vi "PulseGeneratorSetup.vi"(4 "Pulse duration (s)\nif more than one pulse":dbl, 5 "Channel":enum16{"1", "2", "3", "4", "5", "6", "7", "8"}(ring), 6 "Pulses per\nstimulus":u16, 7 "stimulus specifier":T3, 8 "Stimulus\nduration (s)":dbl, 9 "Time between stimuli,\nstart-to-start (s)":dbl, 10 "Number\nof stimuli":u16, 11 "Initial delay (s)":dbl) -> (0 "error IO":errorcluster, 1 "stimulus parameters":T1, 2 "stimulus information":T2, 3 "stimulus specifier":T3)   [LabVIEW 2014]
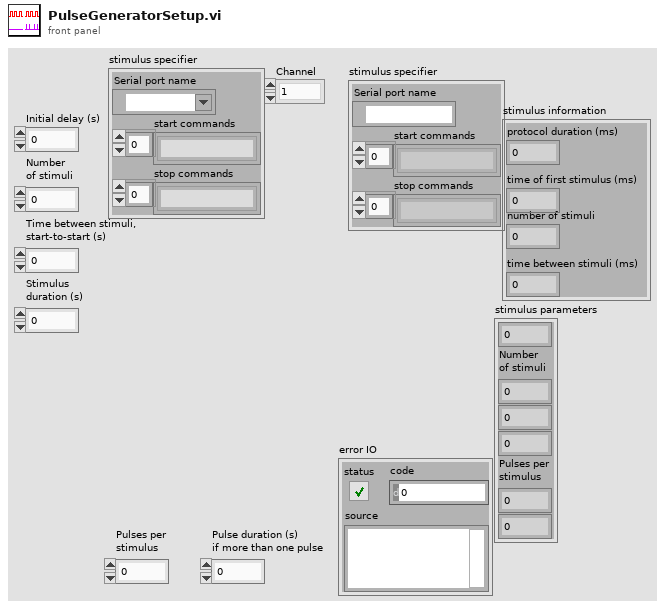
[diagram p1: front panel]
types:
  T1 = cluster{dbl, "Number\nof stimuli":u16, dbl, dbl, "Pulses per\nstimulus":u16, dbl}
  T2 = cluster{"protocol duration (ms)":i64, "time of first stimulus (ms)":i64, "number of stimuli":u16, "time between stimuli (ms)":i64}
  T3 = cluster{"Serial port name":refnum<visa-resource-name>, "start commands":string[], "stop commands":string[]}
  T4 = cluster{i64, "result (ms)":i64, "Number\nof stimuli":u16, i64}
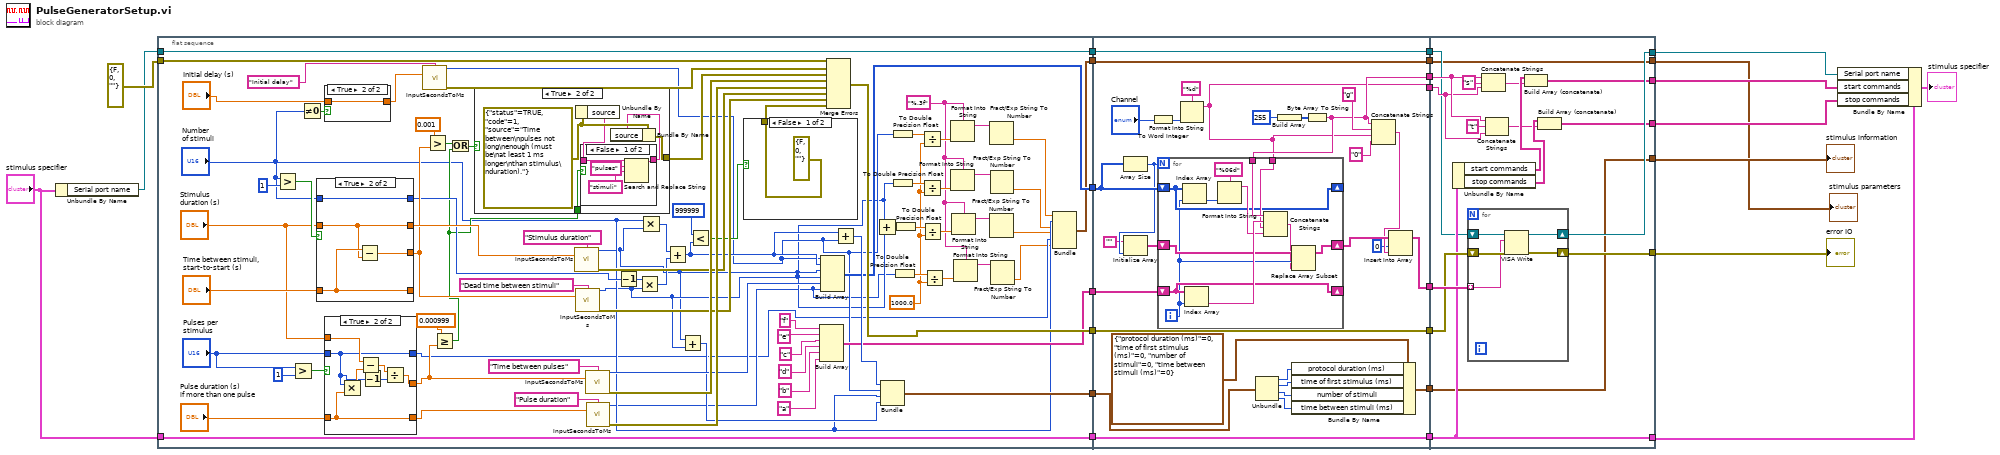
[diagram p0: block diagram]
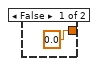
[diagram p2: hidden frame]
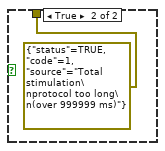
[diagram p3: hidden frame]
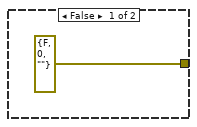
[diagram p4: hidden frame]
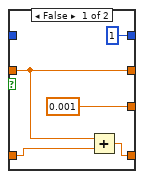
[diagram p6: hidden frame]
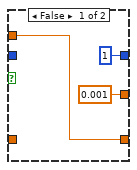
[diagram p7: hidden frame]
diagram:
  n1 = Unbundle By Name("stimulus specifier") -> ("Serial port name"=w11:refnum<visa-resource-name>)
  n2 = flat-sequence {
    tunnel: [w53] -> w9
    tunnel: [w54] -> w8
    tunnel: [w71] -> w7
    tunnel: [w69] -> w6
    tunnel: [w66] -> w5
    tunnel: "stimulus specifier" -> [w69]
    tunnel: errorcluster {"status"=FALSE, "code"=0, "source"=""} ("error constant") -> [w56]
    tunnel: w11 -> [w55]
    tunnel: [w55] -> w4
    tunnel: [w27] -> w3
    tunnel: w9 -> [w169]
    tunnel: w8 -> [w168]
    tunnel: w7 -> [w154]
    tunnel: [w155] -> w26
    tunnel: [w154] -> w25
    tunnel: [w153] -> w24
    tunnel: [w152] -> w23
    tunnel: w6 -> [w151]
    tunnel: [w151] -> w21
    tunnel: w5 -> [w149]
    tunnel: [w144] -> w15
    tunnel: w4 -> [w143]
    tunnel: [w143] -> w10
    tunnel: w3 -> [w142]
    tunnel: [w142] -> w2
    tunnel: w26 -> [w200]
    tunnel: w25 -> [w199]
    tunnel: w24 -> [w196]
    tunnel: w23 -> [w195]
    tunnel: [w194] -> w22
    tunnel: w21 -> [w186]
    tunnel: [w193] -> w19
    tunnel: [w188] -> w18
    tunnel: [w187] -> w17
    tunnel: [w186] -> w20
    tunnel: w15 -> [w185]
    tunnel: [w185] -> w14
    tunnel: w10 -> [w184]
    tunnel: w2 -> [w183]
    tunnel: [w183] -> w1
    frame #0 {
      w40 = 1000.0 ("default (0 I32)")
      w39 = "%.3f"
      n3 = Greater?(x="Number\nof stimuli", y=u16 1) -> (0:w102:bool)
      n4 = Greater?(x="Pulses per\nstimulus", y=u16 1) -> (0:w107:bool)
      n5 = Not Equal To 0?(x="Number\nof stimuli") -> (x != 0?=w59:bool)
      n6 = case shown="True" w102 {
        tunnel: "Time between stimuli,\nstart-to-start (s)" -> [w125 w130]
        tunnel: [w126 w130] -> _
        tunnel: "Number\nof stimuli" -> [_ w131]
        tunnel: "Stimulus\nduration (s)" -> [w124 w129]
        tunnel: [w124 w129] -> w91
        tunnel: [u16 1 ("Number\nof stimuli") w131] -> w84
        tunnel: [0.001 w128] -> w89
        frame False {
          n7 = Add(x=w124, y=w125) -> (x+y=w126:dbl)
        }
        frame True {
          n8 = Subtract(x=w130, y=w129) -> (x-y=w128:dbl)
        }
      }
      n9 = case shown="True" w107 {
        tunnel: "Pulse duration (s)\nif more than one pulse" -> [_ w141]
        tunnel: [w133 w141] -> w95
        tunnel: "Pulses per\nstimulus" -> [_ w137]
        tunnel: [u16 1 ("Pulses per\nstimulus") w137] -> w29
        tunnel: "Stimulus\nduration (s)" -> [w133 w139]
        tunnel: [0.001 w135] -> w64
        frame False {
        }
        frame True {
          n10 = Multiply(x=w137, y=w141) -> (x*y=w140:dbl)
          n11 = Subtract(x=w139, y=w140) -> (x-y=w138:dbl)
          n12 = Decrement(x=w137) -> (x-1=w136:u16)
          n13 = Divide(x=w138, y=w136) -> (x/y=w135:dbl)
        }
      }
      n14 = case shown="True" w59 {
        tunnel: "Initial delay (s)" -> [_ w109]
        tunnel: [0.0 ("Initial delay (s)") w109] -> w57
        frame False {
        }
        frame True {
        }
      }
      n15 = call "InputSecondsToMs.vi"("description"="Initial delay", "value (s)"=w57) -> ("result (ms)"=w38:i64, "error out"=w99:errorcluster)  [unwired: 12 in]
      n16 = Greater?(x=0.001, y=w89) -> (0:w62:bool)
      n17 = Greater Or Equal?(x=0.000999, y=w64) -> (x >= y?=w61:bool)
      n18 = Or(x=w62, y=w61) -> (x .or. y?=w63:bool)
      n19 = case shown="True" w63 {
        tunnel: [errorcluster {"status"=FALSE, "code"=0, "source"=""} ("error constant") w117] -> w97
        tunnel: w61 -> [_ w115]
        frame False {
        }
        frame True {
          w116 = errorcluster {"status"=TRUE, "code"=1, "source"="Time between\npulses not long\nenough (must be\nat least 1 ms longer\nthan stimulus\nduration)."} ("error constant")
          n20 = Unbundle By Name(w116) -> ("source"=w114:string)
          n21 = case shown="False" w115 {
            tunnel: w114 -> [w120 w122]
            tunnel: [w121 w122] -> w113
            frame False {
              n22 = Search and Replace String(input string=w120, search string="pulses", replace string="stimuli" ("replace string (\"\")")) -> (result string=w121:string)  [unwired: 5 in, 3 out]
            }
            frame True {
            }
          }
          n23 = Bundle By Name(cluster=w116, "source"=w113) -> (w117:errorcluster)
        }
      }
      n24 = call "InputSecondsToMs.vi"("description"="Stimulus duration", "value (s)"=w91) -> ("result (ms)"=w33:i64, "error out"=w87:errorcluster)  [unwired: 12 in]
      n25 = call "InputSecondsToMs.vi"("description"="Dead time between stimuli", "value (s)"=w89) -> ("result (ms)"=w34:i64, "error out"=w86:errorcluster)  [unwired: 12 in]
      n26 = call "InputSecondsToMs.vi"("description"="Time between pulses", "value (s)"=w64) -> ("result (ms)"=w78:i64, "error out"=w96:errorcluster)  [unwired: 12 in]
      n27 = call "InputSecondsToMs.vi"("description"="Pulse duration", "value (s)"=w95) -> ("result (ms)"=w31:i64, "error out"=w94:errorcluster)  [unwired: 12 in]
      n28 = Decrement(x=w84) -> (x-1=w85:u16)
      n29 = Multiply(x=w85, y=w34) -> (x*y=w82:i64)
      n30 = Multiply(x="Number\nof stimuli", y=w33) -> (x*y=w83:i64)
      n31 = Add(x=w83, y=w82) -> (x+y=w70:i64)
      n32 = Add(x=w33, y=w34) -> (x+y=w68:i64)
      n33 = Less?(x=i64 999999, y=w70) -> (x < y?=w80:bool)
      n34 = case shown="False" w80 {
        tunnel: [errorcluster {"status"=FALSE, "code"=0, "source"=""} ("error constant") errorcluster {"status"=TRUE, "code"=1, "source"="Total stimulation\nprotocol too long\n(over 999999 ms)"} ("error constant")] -> w79
        frame False {
        }
        frame True {
        }
      }
      n35 = Build Array("f" ("description"), "e" ("description"), "c" ("description"), "d" ("description"), "b" ("description"), "a" ("description")) -> (w54:string[])
      n36 = Build Array(w38, w70, w33, w34, w78, w31) -> (w53:i64[])
      n37 = Merge Errors(w56, w99, w97, w96, w94, w87, w86, w79) -> (w71:errorcluster)
      n38 = Add(x=w70, y=w38) -> (x+y=w67:i64)
      n39 = Add(x=w33, y=w34) -> (x+y=w32:i64)
      n40 = Bundle(w67, "result (ms)"=w38, "Number\nof stimuli"="Number\nof stimuli", w68) -> (w66:T4)  [unwired: 1 in]
      n41 = To Double Precision Float(number=w38) -> (double precision float=w50:dbl)
      n42 = To Double Precision Float(number=w33) -> (double precision float=w47:dbl)
      n43 = To Double Precision Float(number=w31) -> (double precision float=w41:dbl)
      n44 = To Double Precision Float(number=w32) -> (double precision float=w44:dbl)
      n45 = Divide(x=w50, y=w40) -> (x/y=w51:dbl)
      n46 = Divide(x=w47, y=w40) -> (x/y=w48:dbl)
      n47 = Divide(x=w44, y=w40) -> (x/y=w45:dbl)
      n48 = Divide(x=w41, y=w40) -> (x/y=w42:dbl)
      n49 = Format Into String(format string=w39, w51) -> (resulting string=w52:string)  [unwired: 2 in, 1 out]
      n50 = Format Into String(format string=w39, w48) -> (resulting string=w49:string)  [unwired: 2 in, 1 out]
      n51 = Format Into String(format string=w39, w45) -> (resulting string=w46:string)  [unwired: 2 in, 1 out]
      n52 = Format Into String(format string=w39, w42) -> (resulting string=w43:string)  [unwired: 2 in, 1 out]
      n53 = Fract/Exp String To Number(string=w52) -> (number=w37:dbl)  [unwired: 3 in, 1 out]
      n54 = Fract/Exp String To Number(string=w46) -> (number=w30:dbl)  [unwired: 3 in, 1 out]
      n55 = Fract/Exp String To Number(string=w49) -> (number=w35:dbl)  [unwired: 3 in, 1 out]
      n56 = Fract/Exp String To Number(string=w43) -> (number=w28:dbl)  [unwired: 3 in, 1 out]
      n57 = Bundle(w37, "Number\nof stimuli"="Number\nof stimuli", w35, w30, "Pulses per\nstimulus"=w29, w28) -> (w27:T1)  [unwired: 1 in]
    }
    frame #1 {
      n58 = Array Size(array=w169) -> (size(s)=w163:i32)
      n59 = Initialize Array("", w163) -> (w161:string[])
      n60 = To Word Integer(number="Channel") -> (16bit integer=w165:i16)
      n61 = Format Into String(format string="%d", w165) -> (resulting string=w152:string)  [unwired: 2 in, 1 out]
      n62 = Unbundle(w149) -> (w148:i64, "result (ms)"=w147:i64, "Number\nof stimuli"=w146:u16, w145:i64)
      n63 = Build Array(u8 255 ("element")) -> (w166:u8[])
      n64 = Bundle By Name(cluster=T2 {"protocol duration (ms)"=0, "time of first stimulus (ms)"=0, "number of stimuli"=0, "time between stimuli (ms)"=0}, "protocol duration (ms)"=w148, "time of first stimulus (ms)"=w147, "number of stimuli"=w146, "time between stimuli (ms)"=w145) -> (w144:T2)
      n65 = Byte Array To String(unsigned byte array=w166) -> (string=w153:string)
      n66 = for {
        N: w163 -> [_]
        shift-right: [w175] -> _
        shift-left: w169 -> [w175]
        shift-right: [w176] -> _
        shift-left: w168 -> [w176]
        tunnel: w153 -> [w180]
        tunnel: w152 -> [w178]
        shift-right: [w174] -> w160
        shift-left: w161 -> [w173]
        i -> [w172]
        n67 = Index Array(array=w175, index=w172) -> (element=w182:i64)
        n68 = Index Array(array=w176, index=w172) -> (element=w179:string)
        n69 = Format Into String(format string="%06d", w182) -> (resulting string=w177:string)  [unwired: 2 in, 1 out]
        n70 = Concatenate Strings(w180, w179, w178, w177) -> (w171:string)
        n71 = Replace Array Subset(array=w173, new element=w171, index=w172) -> (w174:string[])
      }
      n72 = Concatenate Strings(w153, "g" ("string"), w152, "0" ("string")) -> (w157:string)
      n73 = Insert Into Array(array=w160, index=0, new element=w157) -> (w155:string[])
    }
    frame #2 {
      n74 = Unbundle By Name(w186) -> ("start commands"=w192:string[], "stop commands"=w190:string[])
      n75 = for {
        tunnel: w200 -> [w201] mode=indexing
        shift-right: [w204] -> w193
        shift-left: w184 -> [w205]
        shift-right: [w202] -> w194
        shift-left: w199 -> [w203]
        n76 = VISA Write(VISA resource name=w205, write buffer=w201, error in (no error)=w203) -> (VISA resource name out=w204:refnum<visa-resource-name>, error out=w202:errorcluster)  [unwired: 1 out]
      }
      n77 = Concatenate Strings(w196, "s" ("string"), w195) -> (w191:string)
      n78 = Concatenate Strings(w196, "t" ("string"), w195) -> (w189:string)
      n79 = Build Array (concatenate)(w192, w191) -> (w188:string[])
      n80 = Build Array (concatenate)(w190, w189) -> (w187:string[])
    }
  }
  n81 = Bundle By Name(cluster=w20, "Serial port name"=w19, "start commands"=w18, "stop commands"=w17) -> (→"stimulus specifier":T3)
  "error IO" <- w22
  "stimulus information" <- w14
  "stimulus parameters" <- w1
